vi "Set_Adam_Watchdogs.vi"(1 "Set Watchdogs":bool) -> (0 "Error String":string)   [LabVIEW 2011]
uses:
  Anemometry/Anemometry Sub Vis/Globals/Constants_global.vi
panel:
  out "Day Time":bool
  out "Display":string[][](table)
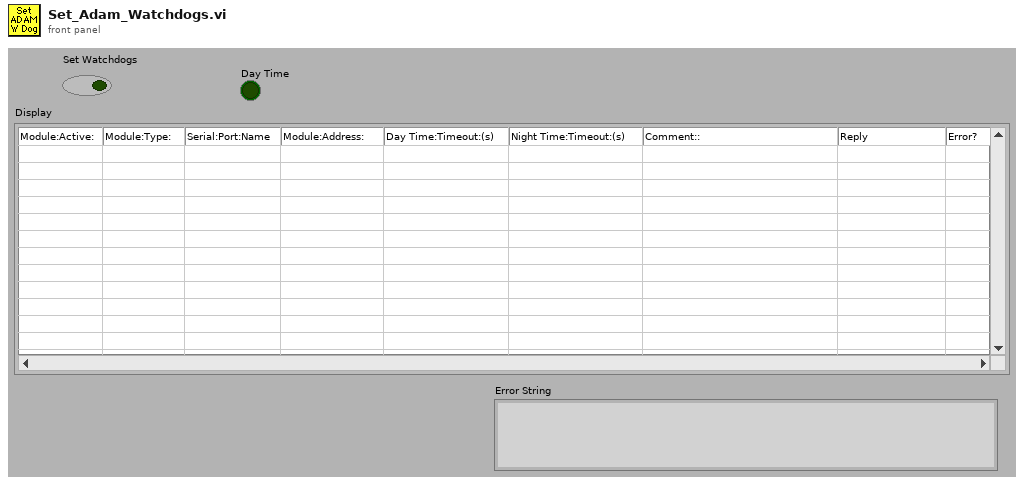
[diagram p1: front panel]
types:
  T1 = typedef "LVDateTimeRec.ctl" = cluster{"fractional second":dbl, "second":i32, "minute":i32, "hour":i32, "day of month":i32, "month":i32, "year":i32, "day of week":i32, "day of year":i32, "DST":i32}
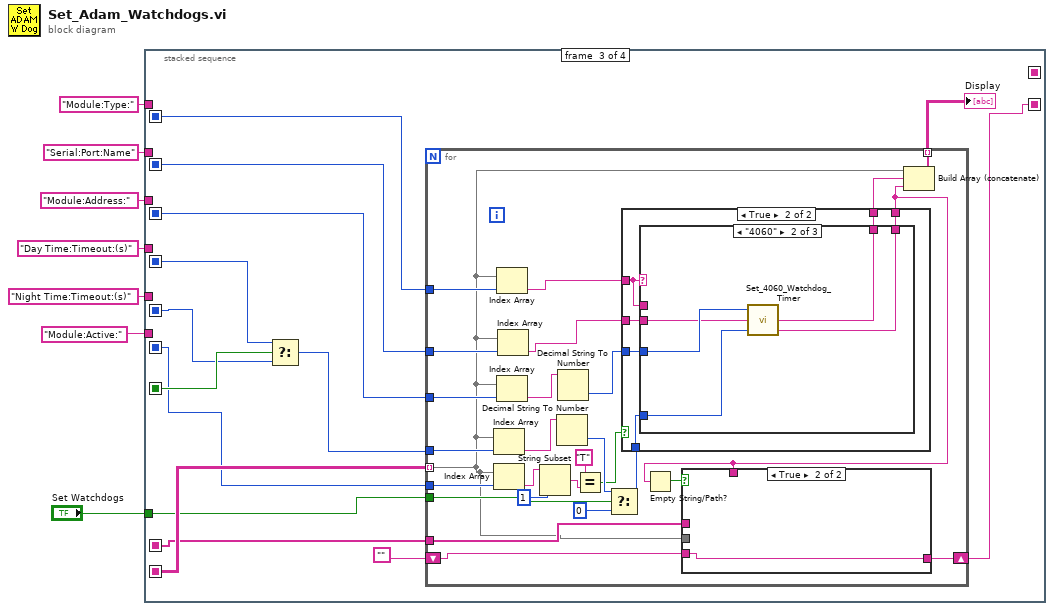
[diagram p0: block diagram]
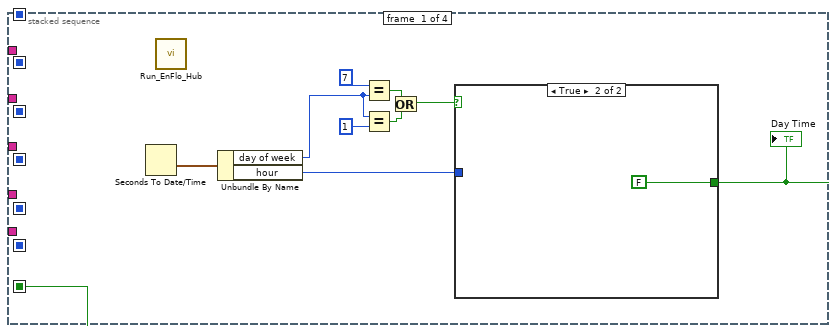
[diagram p2: hidden frame]
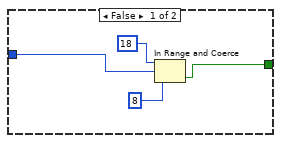
[diagram p3: hidden frame]
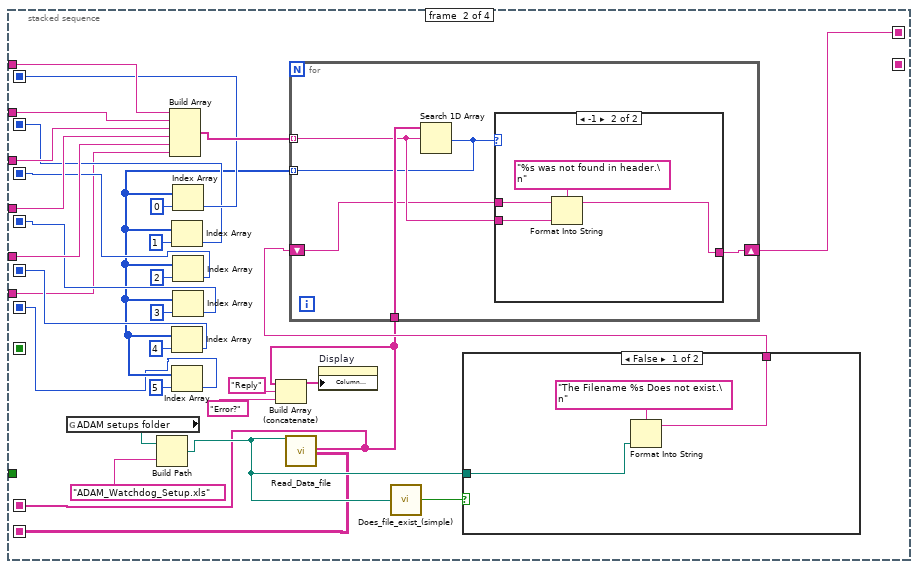
[diagram p4: hidden frame]
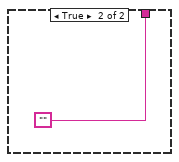
[diagram p5: hidden frame]
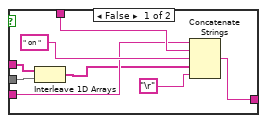
[diagram p7: hidden frame]
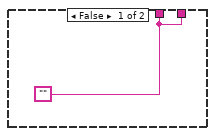
[diagram p8: hidden frame]
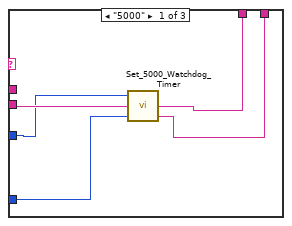
[diagram p9: hidden frame]
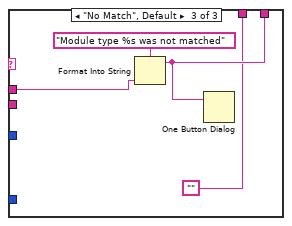
[diagram p10: hidden frame]
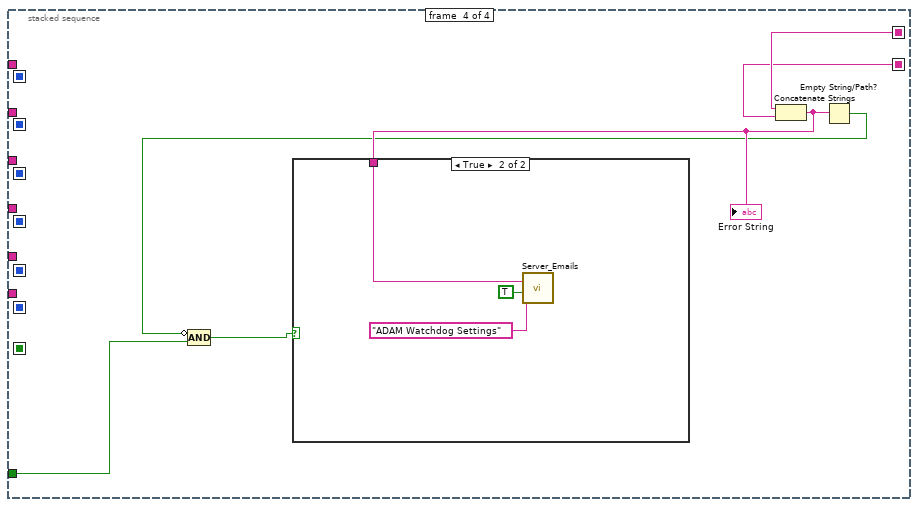
[diagram p11: hidden frame]
diagram:
  n1 = stacked-sequence {
    seq-local: [w8 _ _ _] -> [_ _ w79 _]
    seq-local: [_ w35 _ _] -> [_ _ w77 _]
    seq-local: [_ w34 _ _] -> [_ _ w76 _]
    seq-local: [_ w33 _ _] -> [_ _ w75 _]
    seq-local: [_ w32 _ _] -> [_ _ w74 _]
    seq-local: [_ w31 _ _] -> [_ _ w73 _]
    seq-local: [_ w41 _ _] -> [_ _ _ w143]
    seq-local: [_ w30 _ _] -> [_ _ w78 _]
    seq-local: [_ _ w70 _] -> [_ _ _ w142]
    seq-local: [_ w23 _ _] -> [_ _ w68 _]
    seq-local: [_ w22 _ _] -> [_ _ w67 _]
    tunnel: "Module:Type:" -> [_ w50 _ _]
    tunnel: "Serial:Port:Name" -> [_ w49 _ _]
    tunnel: "Module:Address:" -> [_ w48 _ _]
    tunnel: "Day Time:Timeout:(s)" -> [_ w47 _ _]
    tunnel: "Night Time:Timeout:(s)" -> [_ w46 _ _]
    tunnel: "Set Watchdogs" -> [_ _ w69 w140]
    tunnel: "Module:Active:" -> [_ w26 _ _]
    frame #0 {
      n2 = Seconds To Date/Time() -> (date time rec=w9:T1)  [unwired: 2 in]
      n3 = call "Run_EnFlo_Hub.vi"() -> ()  [unwired: 8 in]
      n4 = Unbundle By Name(w9) -> ("day of week"=w11:i32, "hour"=w16:i32)
      n5 = Equal?(x=7, y=w11) -> (x = y?=w13:bool)
      n6 = Equal?(x=w11, y=1) -> (x = y?=w14:bool)
      n7 = Or(x=w13, y=w14) -> (x .or. y?=w15:bool)
      n8 = case shown="True" w15 {
        tunnel: w16 -> [w20 _]
        tunnel: [w17 FALSE] -> w8
        frame False {
          n9 = In Range and Coerce(upper limit=18, x=w20, lower limit=8) -> (In Range?=w17:bool)  [unwired: 1 out]
        }
        frame True {
        }
      }
      "Day Time" <- w8
    }
    frame #1 {
      n10 = global read "Constants_global.vi" "ADAM setups folder"() -> (w52:path)
      n11 = Build Path(base path=w52, name or relative path="ADAM_Watchdog_Setup.xls") -> (appended path=w43:path)
      n12 = Build Array(w50, w49, w48, w47, w46, w26) -> (w45:string[])
      n13 = call "Read_Data_file.vi"("Results file"=w43) -> ("Ch names Out"=w22:string[], "Channel Values Out"=w30:string[][])  [unwired: 9 in, 8 out]
      n14 = Build Array (concatenate)(w22, "Reply", "Error?" ("element")) -> (w28:string[])
      n15 = property on="Display" class="Tbl (strict)"("Column Headers[]"=w28) -> ()  [unwired: 2 in, 2 out]
      n16 = call "Does_file_exist_(simple).vi"("Pathname"=w43) -> ("exists?"=w44:bool)
      n17 = case shown="False" w44 {
        tunnel: w43 -> [w55 _]
        tunnel: [w53 ""] -> w42
        frame False {
          n18 = Format Into String(format string="The Filename %s Does not exist.\n", w55) -> (resulting string=w53:string)  [unwired: 2 in, 1 out]
        }
        frame True {
        }
      }
      n19 = for {
        tunnel: w22 -> [w61]
        tunnel: w45 -> [w60] mode=indexing
        shift-right: [w58] -> w41
        shift-left: w42 -> [w59]
        tunnel: [w57] -> w24 mode=indexing
        n20 = Search 1D Array(1D array=w61, element=w60) -> (index of element=w57:i32)  [unwired: 1 in]
        n21 = case shown="-1" w57 {
          tunnel: w60 -> [_ w66]
          tunnel: w59 -> [w62 w64]
          tunnel: [w62 w63] -> w58
          frame 0, Default {
          }
          frame -1 {
            n22 = Format Into String(format string="%s was not found in header.\n", initial string=w64, w66) -> (resulting string=w63:string)  [unwired: 1 in, 1 out]
          }
        }
      }
      n23 = Index Array(array=w24, index=1) -> (element=w34:i32)
      n24 = Index Array(array=w24, index=4) -> (element=w31:i32)
      n25 = Index Array(array=w24, index=5) -> (element=w23:i32)
      n26 = Index Array(array=w24, index=0) -> (element=w35:i32)
      n27 = Index Array(array=w24, index=2) -> (element=w33:i32)
      n28 = Index Array(array=w24, index=3) -> (element=w32:i32)
    }
    frame #2 {
      n29 = Select(t=w74, s=w79, f=w73) -> (s? t:f=w72:i32)
      n30 = for {
        tunnel: w78 -> [w84] mode=indexing
        tunnel: w69 -> [w102]
        tunnel: [w97] -> w80 mode=indexing
        tunnel: w77 -> [w96]
        tunnel: w76 -> [w95]
        tunnel: w75 -> [w94]
        tunnel: w72 -> [w93]
        shift-right: [w81] -> w70
        shift-left: "" -> [w82]
        tunnel: w68 -> [w92]
        tunnel: w67 -> [w85]
        n31 = Index Array(array=w84, index=w93) -> (element=w103:string)
        n32 = Index Array(array=w84, index=w92) -> (element=w90:string)
        n33 = Index Array(array=w84, index=w96) -> (element=w107:string)
        n34 = Index Array(array=w84, index=w94) -> (element=w105:string)
        n35 = Index Array(array=w84, index=w95) -> (element=w104:string)
        n36 = String Subset(string=w90, length (rest)=1 ("length (rest)")) -> (substring=w89:string)  [unwired: 1 in]
        n37 = Decimal String To Number(string=w103) -> (number=w101:i32)  [unwired: 2 in, 1 out]
        n38 = Decimal String To Number(string=w105) -> (number=w106:i32)  [unwired: 2 in, 1 out]
        n39 = Equal?(x="T", y=w89) -> (x = y?=w87:bool)
        n40 = Select(t=w101, s=w102, f=0) -> (s? t:f=w99:i32)
        n41 = case shown="True" w87 {
          tunnel: w107 -> [_ w118]
          tunnel: w106 -> [_ w123]
          tunnel: w104 -> [_ w122]
          tunnel: w99 -> [_ w121]
          tunnel: [w117 w120] -> w98
          tunnel: [w117 w119] -> w83
          frame False {
            w117 = ""
          }
          frame True {
            n42 = case shown="\"4060\"" w118 {
              tunnel: w118 -> [_ _ w137]
              tunnel: w123 -> [w127 w133 _]
              tunnel: w122 -> [w128 w132 _]
              tunnel: w121 -> [w126 w131 _]
              tunnel: [w125 w130 ""] -> w120
              tunnel: [w124 w129 w135] -> w119
              frame "5000" {
                n43 = call "Set_5000_Watchdog_Timer.vi"("Watchdog Timer  Seconds"=w126, "Port Name"=w128, "Module Address"=w127) -> ("Comment out"=w124:string, "Reply"=w125:string)  [unwired: 1 out]
              }
              frame "4060" {
                n44 = call "Set_4060_Watchdog_Timer.vi"("Watchdog Timer  Seconds"=w131, "Port Name"=w132, "Module Address"=w133) -> ("Comment out"=w129:string, "Reply"=w130:string)  [unwired: 1 out]
              }
              frame "No Match", Default {
                n45 = Format Into String(format string="Module type %s was not matched", w137) -> (resulting string=w135:string)  [unwired: 2 in, 1 out]
                n46 = One Button Dialog(message=w135) -> ()  [unwired: 1 in, 1 out]
              }
            }
          }
        }
        n47 = Empty String/Path?(string/path=w83) -> (empty?=w86:bool)
        n48 = case shown="True" w86 {
          tunnel: w85 -> [w112 _]
          tunnel: w84 -> [w115 _]
          tunnel: w83 -> [w114 _]
          tunnel: w82 -> [w110 w116]
          tunnel: [w111 w116] -> w81
          frame False {
            n49 = Interleave 1D Arrays(w112, w115) -> (w109:string[])
            n50 = Concatenate Strings(w110, w114, " on ", w109, "\r") -> (w111:string)
          }
          frame True {
          }
        }
        n51 = Build Array (concatenate)(w84, w98, w83) -> (w97:string[])
      }
      "Display" <- w80
    }
    frame #3 {
      n52 = Concatenate Strings(w143, w142) -> (w141:string)
      "Error String" <- w141
      n53 = Empty String/Path?(string/path=w141) -> (empty?=w139:bool)
      n54 = Compound Arithmetic op=AND(invert w139, w140) -> (w138:bool)
      n55 = case shown="True" w138 {
        tunnel: w141 -> [_ w144]
        frame False {
        }
        frame True {
          n56 = call "Server_Emails.vi"("Message"=w144, "Contact All clients?"=TRUE, "Subject"="ADAM Watchdog Settings") -> ()  [unwired: 2 in, 3 out]
        }
      }
    }
  }
